vi "DataGraph_UpdPaneColor.vi"(5 "Display State In":T1, 7 "Graph Enable":bool, 8 "error in (no error)":errorcluster, 9 "Main VI Panel":refnum<vi>, 11 "Pane Array":refnum<vi>[](array[refnum])) -> (0 "error out":errorcluster, 3 "Display State Out":T1)   [LabVIEW 2018, in "DataGraphXControl.xctl"]
uses:
  DataGraphXControl.xctl
  DataGraph_State.ctl
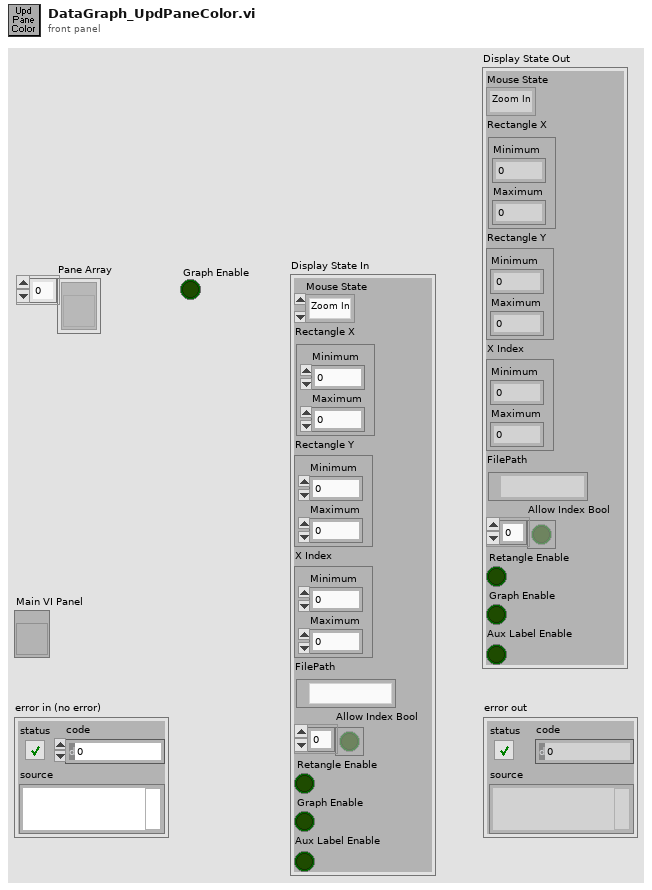
[diagram p1: front panel]
types:
  T1 = typedef "DataGraphXControl.xctl/DataGraph_State.ctl" = cluster{"Mouse State":enum16{"Zoom In", "Select Range"}, "Rectangle X":cluster{"Minimum":dbl, "Maximum":dbl}, "Rectangle Y":cluster{"Minimum":dbl, "Maximum":dbl}, "X Index":cluster{"Minimum":u32, "Maximum":u32}, "FilePath":path, "Allow Index Bool":bool[], "Retangle Enable":bool, "Graph Enable":bool, "Aux Label Enable":bool}
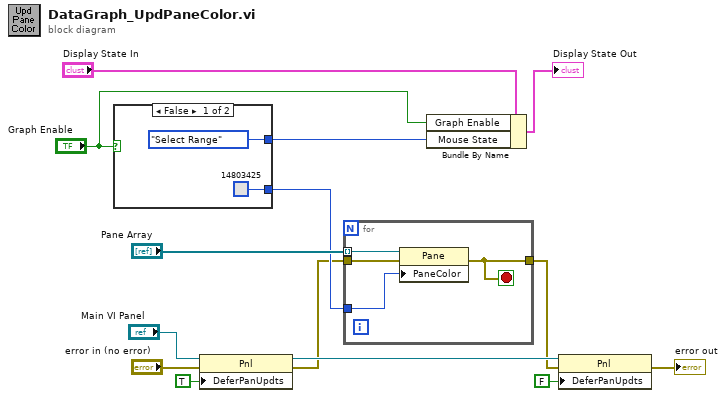
[diagram p0: block diagram]
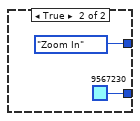
[diagram p2: hidden frame]
diagram:
  n1 = case shown="False" "Graph Enable" {
    tunnel: [u32 14803425 u32 9567230] -> w8
    tunnel: [enum16{"Zoom In", "Select Range"}."Select Range" ("Mouse State") enum16{"Zoom In", "Select Range"}."Zoom In" ("Mouse State")] -> w4
    frame False {
    }
    frame True {
    }
  }
  n2 = property class="Pnl"(reference="Main VI Panel", error in="error in (no error)", "DeferPanUpdts"=TRUE ("Defer Panel Updates")) -> (reference out=w10:refnum<vi>, error out=w7:errorcluster)
  n3 = for {
    tunnel: "Pane Array" -> [w22] mode=indexing
    tunnel: w8 -> [w21]
    tunnel: w7 -> [w20]
    tunnel: [w19] -> w6
    stop <- w19 stop-if-true
    n4 = property class="Pane"(reference=w22, error in=w20, "PaneColor"=w21) -> (error out=w19:errorcluster)  [unwired: 1 out]
  }
  n5 = Bundle By Name(cluster="Display State In", "Graph Enable"="Graph Enable", "Mouse State"=w4) -> (→"Display State Out":T1)
  n6 = property class="Pnl"(reference=w10, error in=w6, "DeferPanUpdts"=FALSE ("Defer Panel Updates")) -> (error out=→"error out":errorcluster)  [unwired: 1 out]
